vi "Filter Correction.vi"(10 "Read Power":dbl, 11 "Power Meter.lvclass In":refnum<class "Power Meter.lvclass">) -> (2 "Corrected Power":dbl, 3 "Power Meter.lvclass Out":refnum<class "Power Meter.lvclass">)   [LabVIEW 2012, in "Power Meter.lvclass"]
doc: "Corrects the power measurement for which filter is being used."
uses:
  Power Meter.lvclass
  Power Meter.lvclass/Power Meter.ctl
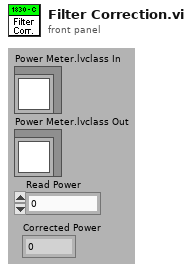
[diagram p1: front panel]
types:
  T1 = typedef "Filters.ctl" = u16
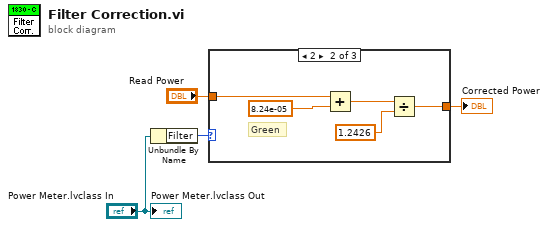
[diagram p0: block diagram]
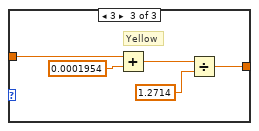
[diagram p3: hidden frame]
diagram:
  n1 = Unbundle By Name("Power Meter.lvclass In") -> ("Filter"=w4:T1)
  n2 = case shown="2" w4 {
    tunnel: "Read Power" -> [w5 w7 w12]
    tunnel: [w5 w6 w11] -> w2
    frame 1, Default {
      # "Orange"
    }
    frame 2 {
      # "Green"
      n3 = Add(x=w7, y=8.24e-05) -> (x+y=w8:dbl)
      n4 = Divide(x=w8, y=1.2426) -> (x/y=w6:dbl)
    }
    frame 3 {
      # "Yellow"
      n5 = Add(x=w12, y=0.0001954) -> (x+y=w13:dbl)
      n6 = Divide(x=w13, y=1.2714) -> (x/y=w11:dbl)
    }
  }
  "Corrected Power" <- w2
  "Power Meter.lvclass Out" <- "Power Meter.lvclass In"
